vi "Sagar C V Universal Gates using Basic Gates.vi"() -> ()   [LabVIEW 2018]
panel:
  in  "?":string
  in  "?":string
  out "NOR GATE USING BASIC GATE":bool
  out "NAND GATE USING BASIC GATE":bool
  in  "B":bool
  in  "A":bool
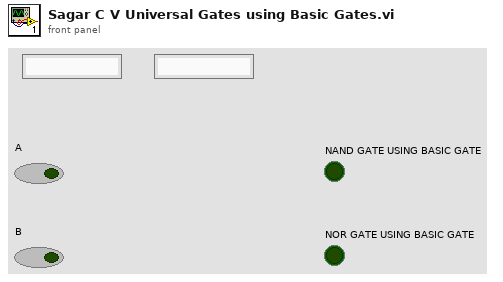
[diagram p1: front panel]
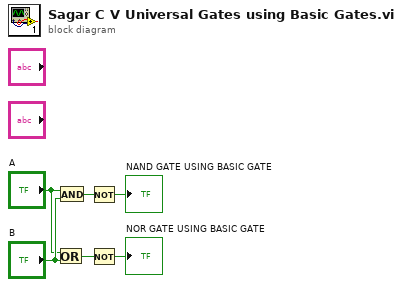
[diagram p0: block diagram]
diagram:
  n1 = Or(x="A", y="B") -> (x .or. y?=w3:bool)
  n2 = And(x="A", y="B") -> (x .and. y?=w4:bool)
  n3 = Not(x=w4) -> (.not. x?=→"NAND GATE USING BASIC GATE":bool)
  n4 = Not(x=w3) -> (.not. x?=→"NOR GATE USING BASIC GATE":bool)
